vi "CANFD Get Bus Error.vi"(9 "pCanBusError":T1, 10 "CANIndex":u8, 11 "DevHandle":i32) -> (1 "pCanBusError out":T1, 3 "function return":i32)   [LabVIEW 2010, in "usb2canfd.lvlib"]
doc: "int WINAPI CANFD_GetBusError(int DevHandle, unsigned char CANIndex, CANFD_BUS_ERROR *pCanBusError);"
uses:
  usb2canfd.lvlib
  USB2XXX/trunk/USB2XXX/USB2XXX/vs2019/Release/USB2XXX.dll
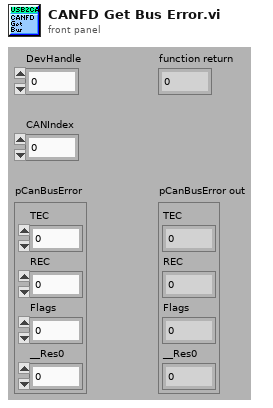
[diagram p1: front panel]
types:
  T1 = cluster{"TEC":u8, "REC":u8, "Flags":u8, "__Res0":u8}
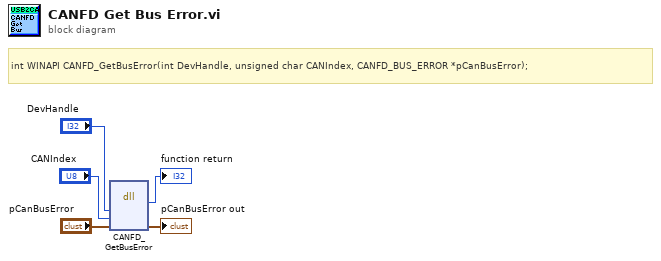
[diagram p0: block diagram]
diagram:
  # "int WINAPI CANFD_GetBusError(int DevHandle, unsigned char CANIndex, CANFD_BUS_ERROR *pCanBusError);"
  n1 = dll-call lib="E:/Projects/USB2XXX/trunk/USB2XXX/USB2XXX/vs2019/Release/USB2XXX.*" fn="CANFD_GetBusError"("DevHandle"="DevHandle", "CANIndex"="CANIndex", "pCanBusError"="pCanBusError") -> (→"function return":i32, "pCanBusError"=→"pCanBusError out":T1)  [unwired: 5 in, 2 out]
